vi "Test Get Summary of Method with Multiple Assertions.vi"(8 "error in (no error)":errorcluster, 11 "Result Model Result Recording Test in":refnum<class "Result Model Result Recording Test.lvclass">) -> (0 "error out":errorcluster, 3 "Result Model Result Recording Test out":refnum<class "Result Model Result Recording Test.lvclass">)   [LabVIEW 2020, in "Result Model Result Recording Test.lvclass"]
uses:
  Result Model Result Recording Test.lvclass
  C:/Program Files (x86)/National Instruments/LabVIEW 2020/vi.lib/Astemes/LUnit/Test Case.lvclass
  Core/Result/Result.ctl
  Core/Result/Status.ctl
  Core/Result/Type.ctl
  <vilib>/Astemes/LUnit/Test Case.lvclass/Test Case.ctl
  865a11a4-746d-41de-93c1-4db6b0010296.vi
  <vilib>/Astemes/LUnit/Palette/Pass.vi
  <vilib>/Astemes/LUnit/Palette/Fail.vi
  <vilib>/Astemes/LUnit/Compare Variants.vi
  <vilib>/Astemes/LUnit/Describe Comparison.vi
  <vilib>/Astemes/LUnit/Set Assertion Type.vi
  <vilib>/Astemes/LUnit/Add test result.vi
  <vilib>/Astemes/LUnit/Variant to string.vi
  <vilib>/Astemes/LUnit/LUnit Record Assertion Result.vi
  <vilib>/Astemes/LUnit/LUnit Aggregate Assertion Results.vi
  <vilib>/Astemes/LUnit/Method Result/LUnit Merge Status.vi
  <vilib>/Astemes/LUnit/LUnit Concatenate result strings.vi
  <vilib>/Utility/Data Type/Get Type Information.vi
  <vilib>/Utility/LVClass/Get LV Class Name.vi
  Framework/Result Model/Result Model.lvclass
  Core/Result/Result.lvlib
panel:
  in  "String":string="Assertions evaluated: 1\r\nTest method result: Failed\nExecution time: 0.009\n \n=============Assertions=================\nFail: Failed\nDescription:\nMessage\n\nPass: Passed\nDescription:\nMessage"
  out "Summary":string
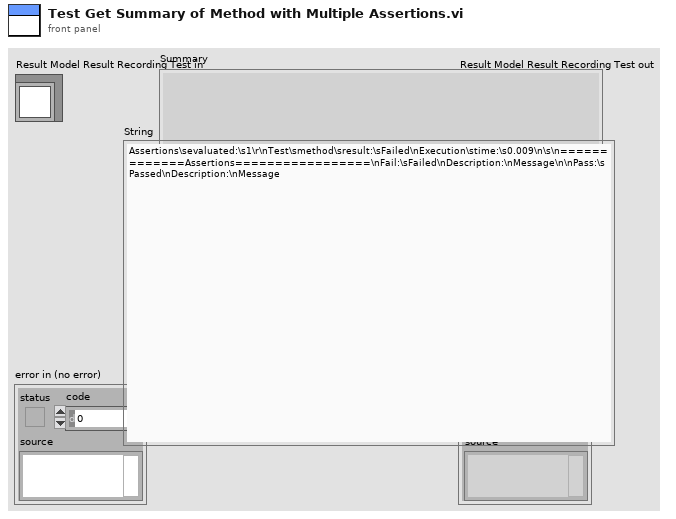
[diagram p1: front panel]
types:
  T1 = typedef "Result.lvlib/Result.ctl" = cluster{"Name":string, "Message":string, "Description":string, "Status":T2, "Result Type":T3, "Execution Time":dbl}
  T2 = typedef "Result.lvlib/Status.ctl" = enum16{"", "Passed", "Failed", "Error", "Skipped", "Setup Error", "Broken", "Teardown Error"}
  T3 = typedef "Result.lvlib/Type.ctl" = enum16{"Method", "Case", "Suite", "Pass", "Fail", "Skip", "Pass if", "Fail if", "Pass if Error", "Fail if Error", "Pass if Equal", "Fail if Equal"}
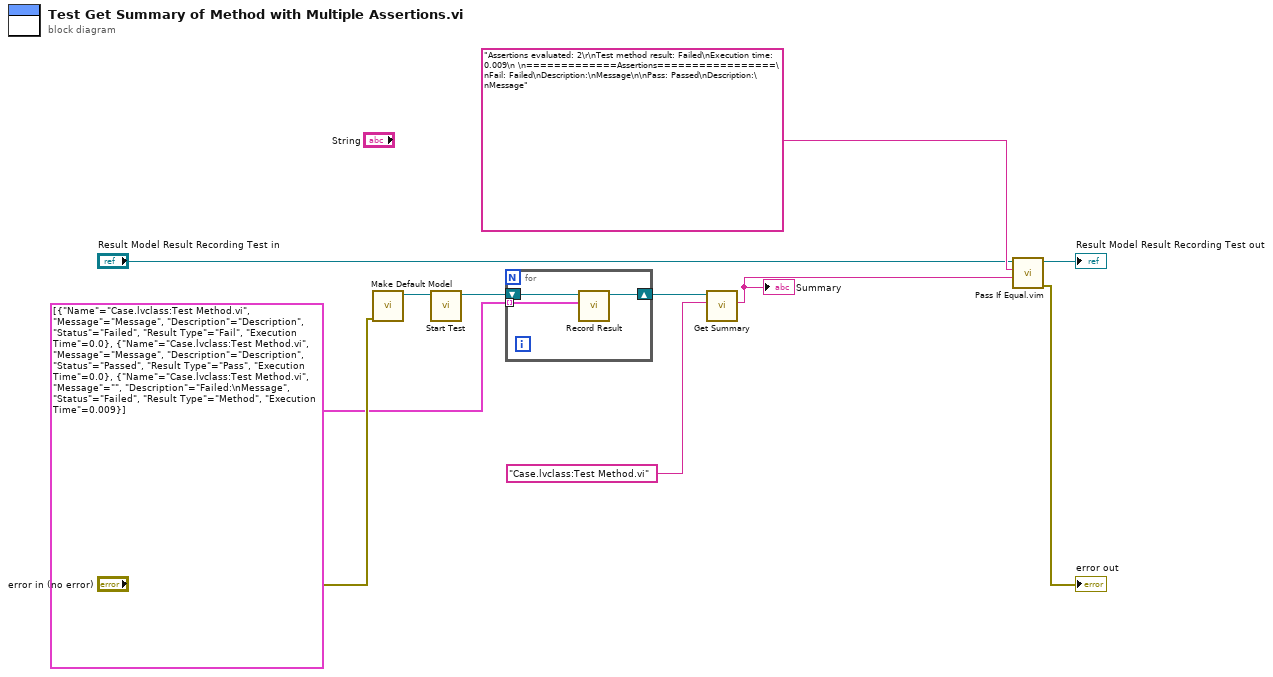
[diagram p0: block diagram]
diagram:
  n1 = call "Make Default Model.vi"("error in (no error)"="error in (no error)") -> ("Result Model out"=w8:refnum<class "Result Model.lvclass">)  [unwired: 9 in, 1 out]
  n2 = call "Start Test.vi"("Result Model In"=w8) -> ("Result Model Out"=w7:refnum<class "Result Model.lvclass">)  [unwired: 10 in]
  n3 = for {
    tunnel: T1[] [{"Name"="Case.lvclass:Test Method.vi", "Message"="Message", "Description"="Description", "Status"=enum."Failed", "Result Type"=enum."Fail", "Execution Time"=0.0}, {"Name"="Case.lvclass:Test Method.vi", "Message"="Message", "Description"="Description", "Status"=enum."Passed", "Result Type"=enum."Pass", "Execution Time"=0.0}, {"Name"="Case.lvclass:Test Method.vi", "Message"="", "Description"="Failed:\nMessage", "Status"=enum."Failed", "Result Type"=enum."Method", "Execution Time"=0.009}] ("Results") -> [w12] mode=indexing
    shift-right: [w13] -> w6
    shift-left: w7 -> [w14]
    n4 = call "Record Result.vi"("Results"=w12, "Result Model in"=w14) -> ("Result Model out"=w13:refnum<class "Result Model.lvclass">)  [unwired: 9 in]
  }
  n5 = call "Get Summary.vi"("Item"="Case.lvclass:Test Method.vi", "Result Model In"=w6) -> ("Summary"=w3:string)  [unwired: 9 in]
  "Summary" <- w3
  n6 = call "Pass If Equal.vim"("Actual"=w3, "Expected"="Assertions evaluated: 2\r\nTest method result: Failed\nExecution time: 0.009\n \n=============Assertions=================\nFail: Failed\nDescription:\nMessage\n\nPass: Passed\nDescription:\nMessage", "LUnit Test Case In"="Result Model Result Recording Test in") -> ("error out"=→"error out":errorcluster, "LUnit Test Case Out"=→"Result Model Result Recording Test out":refnum<class "Result Model Result Recording Test.lvclass">)  [unwired: 7 in]
